vi "Vision Research Phantom Series PhFile PhGetCineAuxData.vi"(1 "CH in":u64, 2 "ImageNumber":i32, 3 "SelectionCode":enum16{"GAD_TIME", "GAD_EXPOSURE"}(ring), 4 "DataSize":u32, 5 "Error In (no error)":errorcluster) -> (15 "CH out":u64, 17 "pData (TIME64)":T1[](array[typedef]) {"fractions" format="%32.0f"}, 18 "pData (UINT)":u32[](array[numeric]), 19 "Error Out":errorcluster)   [LabVIEW 2013, in "VRI.lvlib"]
doc: "PhFile.dll\n\nPhGetCineAuxData\nHRESULT PhGetCineAuxData(CINEHANDLE CH, INT ImageNumber, UINT SelectionCode, UINT DataSize, PVOID pData);\n\nParameters Description\nCH(in) Handle of the cine.\nImageNumber(in) The number of the cine image.\nSelectionCode(in) GAD_TIME – in order to take the time of acquisition fora specified image from the cine.\n GAD_EXPOSURE – to take the exposure of an image\nDataSize(in) Size of the data structure that is returned in pData.\npData(out) May be time (TIME64) or exposure (UINT).\nReturn HRESULT (0 = Ok)\n ERR_BADCINE – Cine handle was not initialized.\nComments This function returns in pTime an array of time moments. pTime[0] is the moment of \n acquisition of the first image.\n\nWritten by:\nBLOOMY CONTROLS, INC\nWINDSOR, CT 06095, USA\n860-298-9925\nwww.bloomy.com\nV1.0.0\nMay, 2004"
uses:
  VRI.lvlib
  _Type Defs/PHCon Time64.ctl
  Phantom DLLs/PhFile.dll
panel:
  # "For instructions on the use of this VI, press Ctrl+H to display the help window and move the mouse over the icon, controls, and indicators"
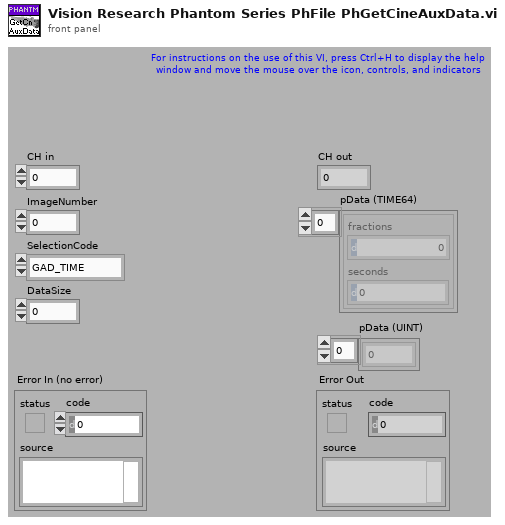
[diagram p1: front panel]
types:
  T1 = typedef "VRI.lvlib/PHCon Time64.ctl" = cluster{"fractions":u32, "seconds":u32}
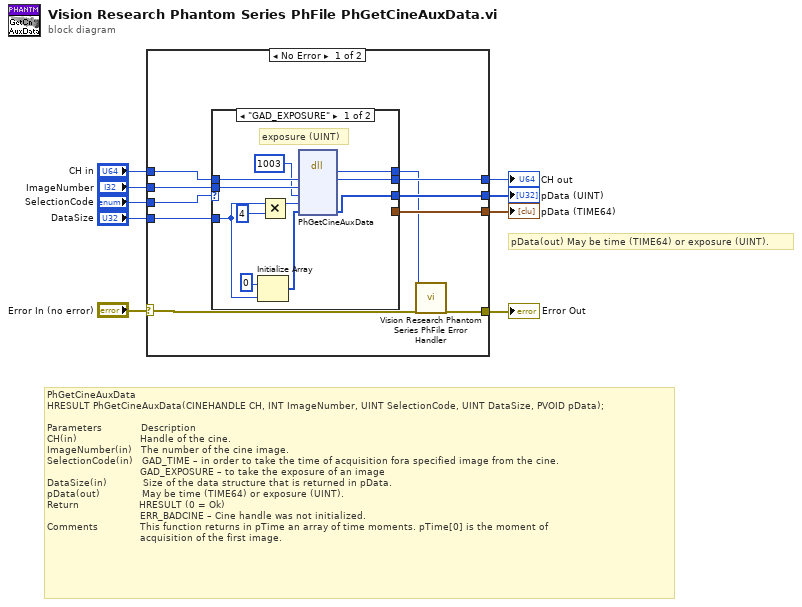
[diagram p0: block diagram]
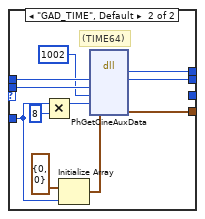
[diagram p2: hidden frame]
diagram:
  # "pData(out) May be time (TIME64) or exposure (UINT)."
  # "PhGetCineAuxData\nHRESULT PhGetCineAuxData(CINEHANDLE CH, INT ImageNumber, UINT SelectionCode, UINT DataSize, PVOID pData);\n\nParameters             Description\nCH(in)                     Handle of the cine.\nImageNumber(in)   The number of the cine image.\nSelectionCode(in)   GAD_TIME – in order to take the time of acquisition fora specified image from the cine.\n                               GAD_EXPOSURE – to take the exposure of an image\nDataSize(in)            Size of the data structure that is returned in pData.\npData(out)              May be time (TIME64) or exposure (UINT).\nReturn                    HRESULT (0 = Ok)\n                               ERR_BADCINE – Cine handle was not initialized.\nComments              This function returns in pTime an array of time moments. pTime[0] is the moment of \n                               acquisition of the first image."
  n1 = case shown="No Error" "Error In (no error)" {
    selector: "Error In (no error)" -> [w19 w43]
    tunnel: [w18 w43] -> w8
    tunnel: [w17 w42] -> w7
    tunnel: "CH in" -> [w16 w42]
    tunnel: "ImageNumber" -> [w15 _]
    tunnel: "DataSize" -> [w14 _]
    tunnel: "SelectionCode" -> [w13 _]
    tunnel: [w12 _] -> w2
    tunnel: [w11 _] -> w1
    frame No Error {
      n2 = case shown="\"GAD_EXPOSURE\"" w13 {
        tunnel: [w30 w41] -> w10
        tunnel: [w28 w39] -> w17
        tunnel: w16 -> [w29 w38]
        tunnel: w15 -> [w27 w37]
        tunnel: w14 -> [w25 w35]
        tunnel: [_ w36] -> w12
        tunnel: [w26 _] -> w11
        frame "GAD_EXPOSURE" {
          # "exposure (UINT)"
          n3 = Initialize Array(u32 0, w25) -> (w24:u32[])
          n4 = Multiply(x=w25, y=u32 4) -> (x*y=w22:u32)
          n5 = dll-call lib="C:/Projects/SDK/32-bit/Vision Research Phantom Series Labview Driver/Phantom DLLs/PhFile.dll" fn="PhGetCineAuxData"("CH"=w29, "ImageNumber"=w27, "SelectionCode"=u32 1003, "DataSize"=w22, "pData"=w24) -> ("HRESULT"=w30:i32, "CH"=w28:u64, "pData"=w26:u32[])  [unwired: 5 in, 3 out]
        }
        frame "GAD_TIME", Default {
          # "(TIME64)"
          n6 = Multiply(x=w35, y=u32 8) -> (x*y=w33:u32)
          n7 = Initialize Array(T1 {"fractions"=0, "seconds"=0} ("Time64"), w35) -> (w40:T1[])
          n8 = dll-call lib="C:/Projects/SDK/32-bit/Vision Research Phantom Series Labview Driver/Phantom DLLs/PhFile.dll" fn="PhGetCineAuxData"("CH"=w38, "ImageNumber"=w37, "SelectionCode"=u32 1002, "DataSize"=w33, "pData"=w40) -> ("HRESULT"=w41:i32, "CH"=w39:u64, "pData"=w36:T1[])  [unwired: 5 in, 3 out]
        }
      }
      n9 = call "Vision Research Phantom Series PhFile Error Handler.vi"("Error Code (0)"=w10, "Error In (no error)"=w19) -> ("Error Out"=w18:errorcluster)  [unwired: 17 out]
    }
    frame Error {
    }
  }
  "Error Out" <- w8
  "CH out" <- w7
  "pData (TIME64)" <- w2
  "pData (UINT)" <- w1
